vi "get scanivalve config filepath from channel config filepath.vi"(11 "channel config file":path) -> (3 "scanivalve config file":path)   [LabVIEW 2018]
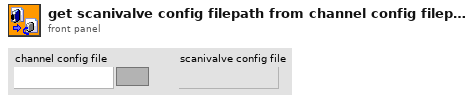
[diagram p1: front panel]
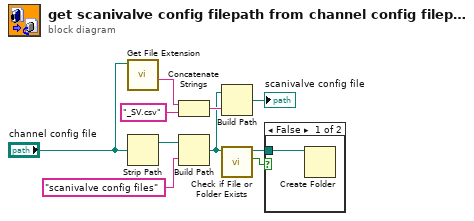
[diagram p0: block diagram]
diagram:
  n1 = call <vilib>:"Get File Extension.vi"("file"="channel config file") -> ("filename without extension"=w1:string)  [unwired: 6 in, 4 out]
  n2 = Strip Path(path="channel config file") -> (stripped path=w5:path)  [unwired: 1 out]
  n3 = Concatenate Strings(w1, "_SV.csv" ("string")) -> (w8:string)
  n4 = Build Path(base path=w5, name or relative path="scanivalve config files") -> (appended path=w4:path)
  n5 = Build Path(base path=w4, name or relative path=w8) -> (appended path=→"scanivalve config file":path)
  n6 = call <vilib>:"Check if File or Folder Exists.vi"("path"=w4) -> ("file or folder exists?"=w3:bool, "dup path"=w2:path)  [unwired: 8 in, 1 out]
  n7 = case shown="False" w3 {
    tunnel: w2 -> [w11 _]
    frame False {
      n8 = Create Folder(path (use dialog)=w11) -> ()  [unwired: 2 in, 3 out]
    }
    frame True {
    }
  }
